vi "LabVIEWRTControlStartupVI.vi"() -> ()   [LabVIEW 2020]
doc: "This example demonstrates a command based communication architecture using TCP. It shows a protocol for packaging and parsing data while minimizing network traffic. Refer to the National Instruments Web site at ni.com/info and enter the info code \"commtcp\" for more information about this command based communication architecture."
uses:
  Control 2.ctl
  ChannelCommand.ctl
  Control 1.ctl
  WaveType.ctl
  MoterEnable.ctl
  <instrlib>/vmic5565/labview-user.lib/VMIC/VMIC 5565 Reflective Memory.llb/VMIC Reference.ctl
  <vilib>/Platform/TimedLoop/XDataNode/timing_clust.ctl
  <vilib>/Platform/TimedLoop/XDataNode/nitl_modes.ctl
  <vilib>/Platform/TimedLoop/XDataNode/wakeup.ctl
  <vilib>/DAQmx/write.llb/DAQmx Write (Analog 1D DBL NChan 1Samp).vi
  <vilib>/DAQmx/write.llb/DAQmx Write (Digital 1D Bool NChan 1Samp 1Line).vi
  <instrlib>/vmic5565/labview-user.lib/VMIC/VMIC 5565 Reflective Memory.llb/VMIC Write (U32).vi
  <vilib>/DAQmx/miscellaneous.llb/DAQmx Fill In Error Info.vi
  <instrlib>/vmic5565/labview-user.lib/VMIC/VMIC 5565 Reflective Memory.llb/VMIC Read (U8).vi
  <vilib>/Platform/TimedLoop/XDataNode/XDataNode.xnode
  <vilib>/Platform/TimedLoop/XDataNode/XDNodeRunTimeDep.lvlib
  <vilib>/real-time/NI_Real-Time Libraries.lvlib
  <vilib>/NI_Real-Time Target Support.lvlib
  <vilib>/real-time/rtutility.llb/RT Restart Target (Self).vi
panel:
  out "输出数组":dbl[](array[numeric])
  out "AngleSample":dbl[](array[numeric])
  out "周期":i64
  out "error out 19":errorcluster caption="错误输出"
  out "error out 18":errorcluster caption="错误输出"
  out "error out 17":errorcluster caption="错误输出"
  out "延迟完成？[i-1]":bool
  out "超时":i32
  out "error out 16":errorcluster caption="错误输出"
  out "error out 15":errorcluster caption="错误输出"
  out "error out 14":errorcluster caption="错误输出"
  out "error out 13":errorcluster caption="错误输出"
  out "error out 3":errorcluster caption="错误输出"
  out "dt":dbl
  out "ResetPosition":dbl[](array[numeric])
  out "Protect":bool
  out "error out 12":errorcluster caption="错误输出"
  out "error out 11":errorcluster caption="error out"
  out "error out 10":errorcluster caption="error out"
  out "error out 9":errorcluster caption="error out"
  out "上传数组":dbl[](array[numeric])
  out "VMIC write":sgl[](array[numeric])
  out "6612counterTask 5":refnum<k21>
  out "ResetAforce":dbl[](array[numeric])
  out "6612counterTask 4":refnum<k21>
  out "6612counterTask 3":refnum<k21>
  out "6612counterTask 2":refnum<k21> caption="任务输出"
  out "6612counterTask":refnum<k21>
  out "x与y? 4":bool[](array[boolean])
  out "VMIC reference":T1
  out "PXI6363IO":refnum<k21>
  out "error out 6":errorcluster caption="error out"
  out "error out 4":errorcluster
  out "Command Type":i32
  out "Msg Head":string
  out "error out":errorcluster caption="错误输出"
  out "长度 3":i32
  out "长度 2":i32
  out "长度":i32
  out "connection ID":refnum<k5> caption="连接ID"
  out "6363Task":refnum<k21> caption="任务输出"
  out "加速度信号":dbl[](array[numeric])
  out "轴向力":dbl[](array[numeric])
  out "T_outrange":bool[](array[boolean])
  out "error out 8":errorcluster caption="error out"
  out "error out 7":errorcluster caption="error out"
  out "error out 5":errorcluster caption="错误输出"
  out "TorqueSampledata 2":dbl[](array[numeric])
  out "command out 2":dbl[](array[numeric])
  out "Wave out 2":dbl[](array[numeric])
  out "type out":dbl[](array[numeric])
  out "Enable":bool[](array[boolean])
  out "StartChannelReset":bool[](array[boolean])
  out "retorquedata2":dbl[](array[numeric])
  out "output 4":dbl[](array[numeric])
  out "TestLoops 2":i32
  out "ResetAngle":dbl[](array[numeric])
  out "ResetTorque":dbl[](array[numeric])
  out "error out 2":errorcluster
  in  "Exit":bool
  out "ControlPara":dbl[][](array[numeric])
  out "ChannelSetArray":T2 {"Enable" items=["不使能", "使能"]; "Wave" items=["0指令", "正弦波", "方波", "三角波", "常值", "波形数据", "白噪声", "正弦扫频", "梯度加载", "VMIC"]; "ChannelType" items=["标准波形跟踪"=1, "扫频测试"=2, "消除多余力"=3, "梯度加载"=4, "载荷谱跟踪"=5, "模拟输入跟踪"=9]; "ChannelStatus" items=["通道关", "位置通道", "加载通道"]}
  out "Stop":bool
  out "iCommand":i32
  out "TestLoops":i32
  out "PXI6738DATask":refnum<k21>
  out "Data array":dbl[][](array[numeric])
  out "error  out":errorcluster
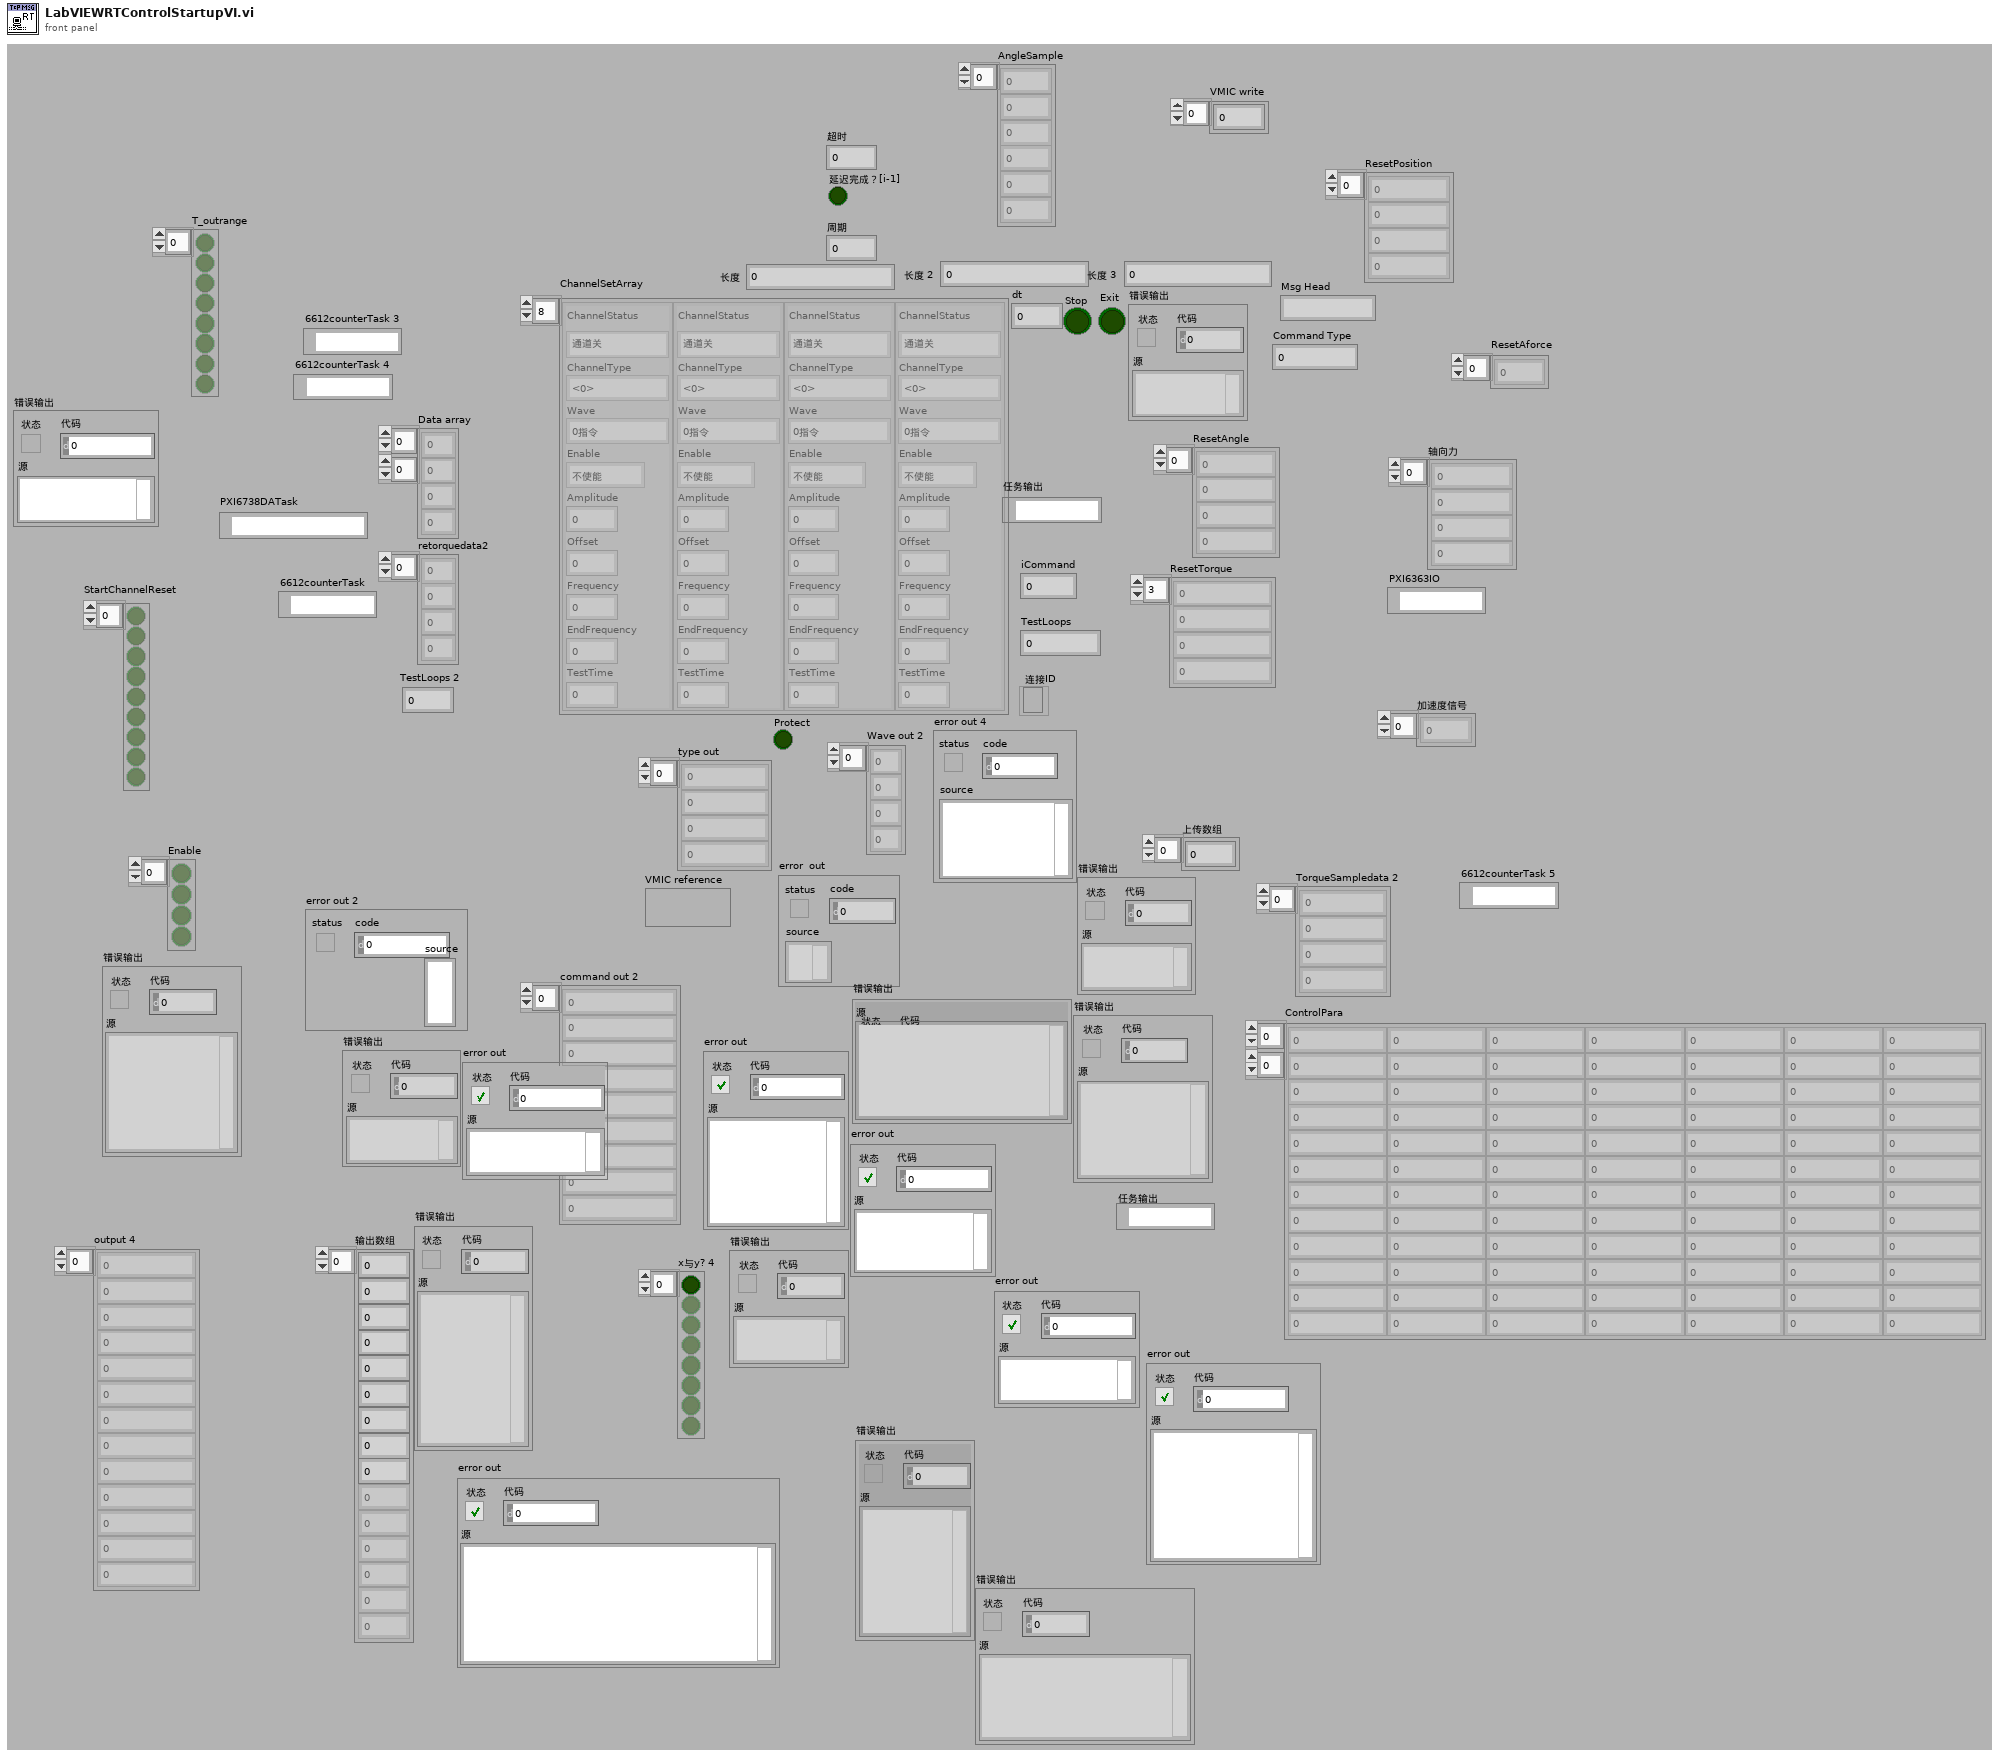
[diagram p1: front panel]
types:
  T1 = typedef "VMIC Reference.ctl" = variant
  T2 = typedef "Control 2.ctl" = T3[]
  T3 = typedef "ChannelCommand.ctl" = cluster{"ChannelStatus":T4, "ChannelType":i32, "Wave":T5, "Enable":T6, "Amplitude":dbl, "Offset":dbl, "Frequency":dbl, "EndFrequency":dbl, "TestTime":dbl}
  T4 = typedef "Control 1.ctl" = i32
  T5 = typedef "WaveType.ctl" = i32
  T6 = typedef "MoterEnable.ctl" = u16
  T7 = typedef "XDNodeRunTimeDep.lvlib/timing_clust.ctl" = cluster{"Expected End [f-1]":u64, "Actual End [f-1]":u64, "Finished Late? [f-1]":bool, "Expected End [i-1]":u64, "Actual End [i-1]":u64, "Finished Late? [i-1]":bool, "Expected Start [i]":u64, "Actual Start [i]":u64, "Expected Start [f]":u64, "Actual Start [f]":u64, "Source Name":string, "Structure Name":string, "Period":i64, "Deadline":i64, "Offset":i64, "Start":i64, "Priority":i32, "Timeout":i32, "Mode":T8, "Wakeup Reason":T9, "Error":errorcluster, "Source Type":string, "Secondary Source Type":string, "Global End Time":u64, "Global Start Time":u64, "Frame Duration":u64, "Iteration Duration":u64, "Assigned CPU":i32, "I/O Scan Engine Mode":u32}
  T8 = typedef "XDNodeRunTimeDep.lvlib/nitl_modes.ctl" = enum32{"No Change", "Process missed periods, maintain original phase", "Discard missed periods, maintain original phase", "Process missed periods, ignore original phase", "Discard missed periods, ignore original phase"}
  T9 = typedef "XDNodeRunTimeDep.lvlib/wakeup.ctl" = enum32{"Normal", "Aborted", "Asynchronous wakeup", "Timing source error", "Timed loop error", "Timeout"}
  T10 = enum16{"big-endian, network order", "native, host order", "little-endian"}
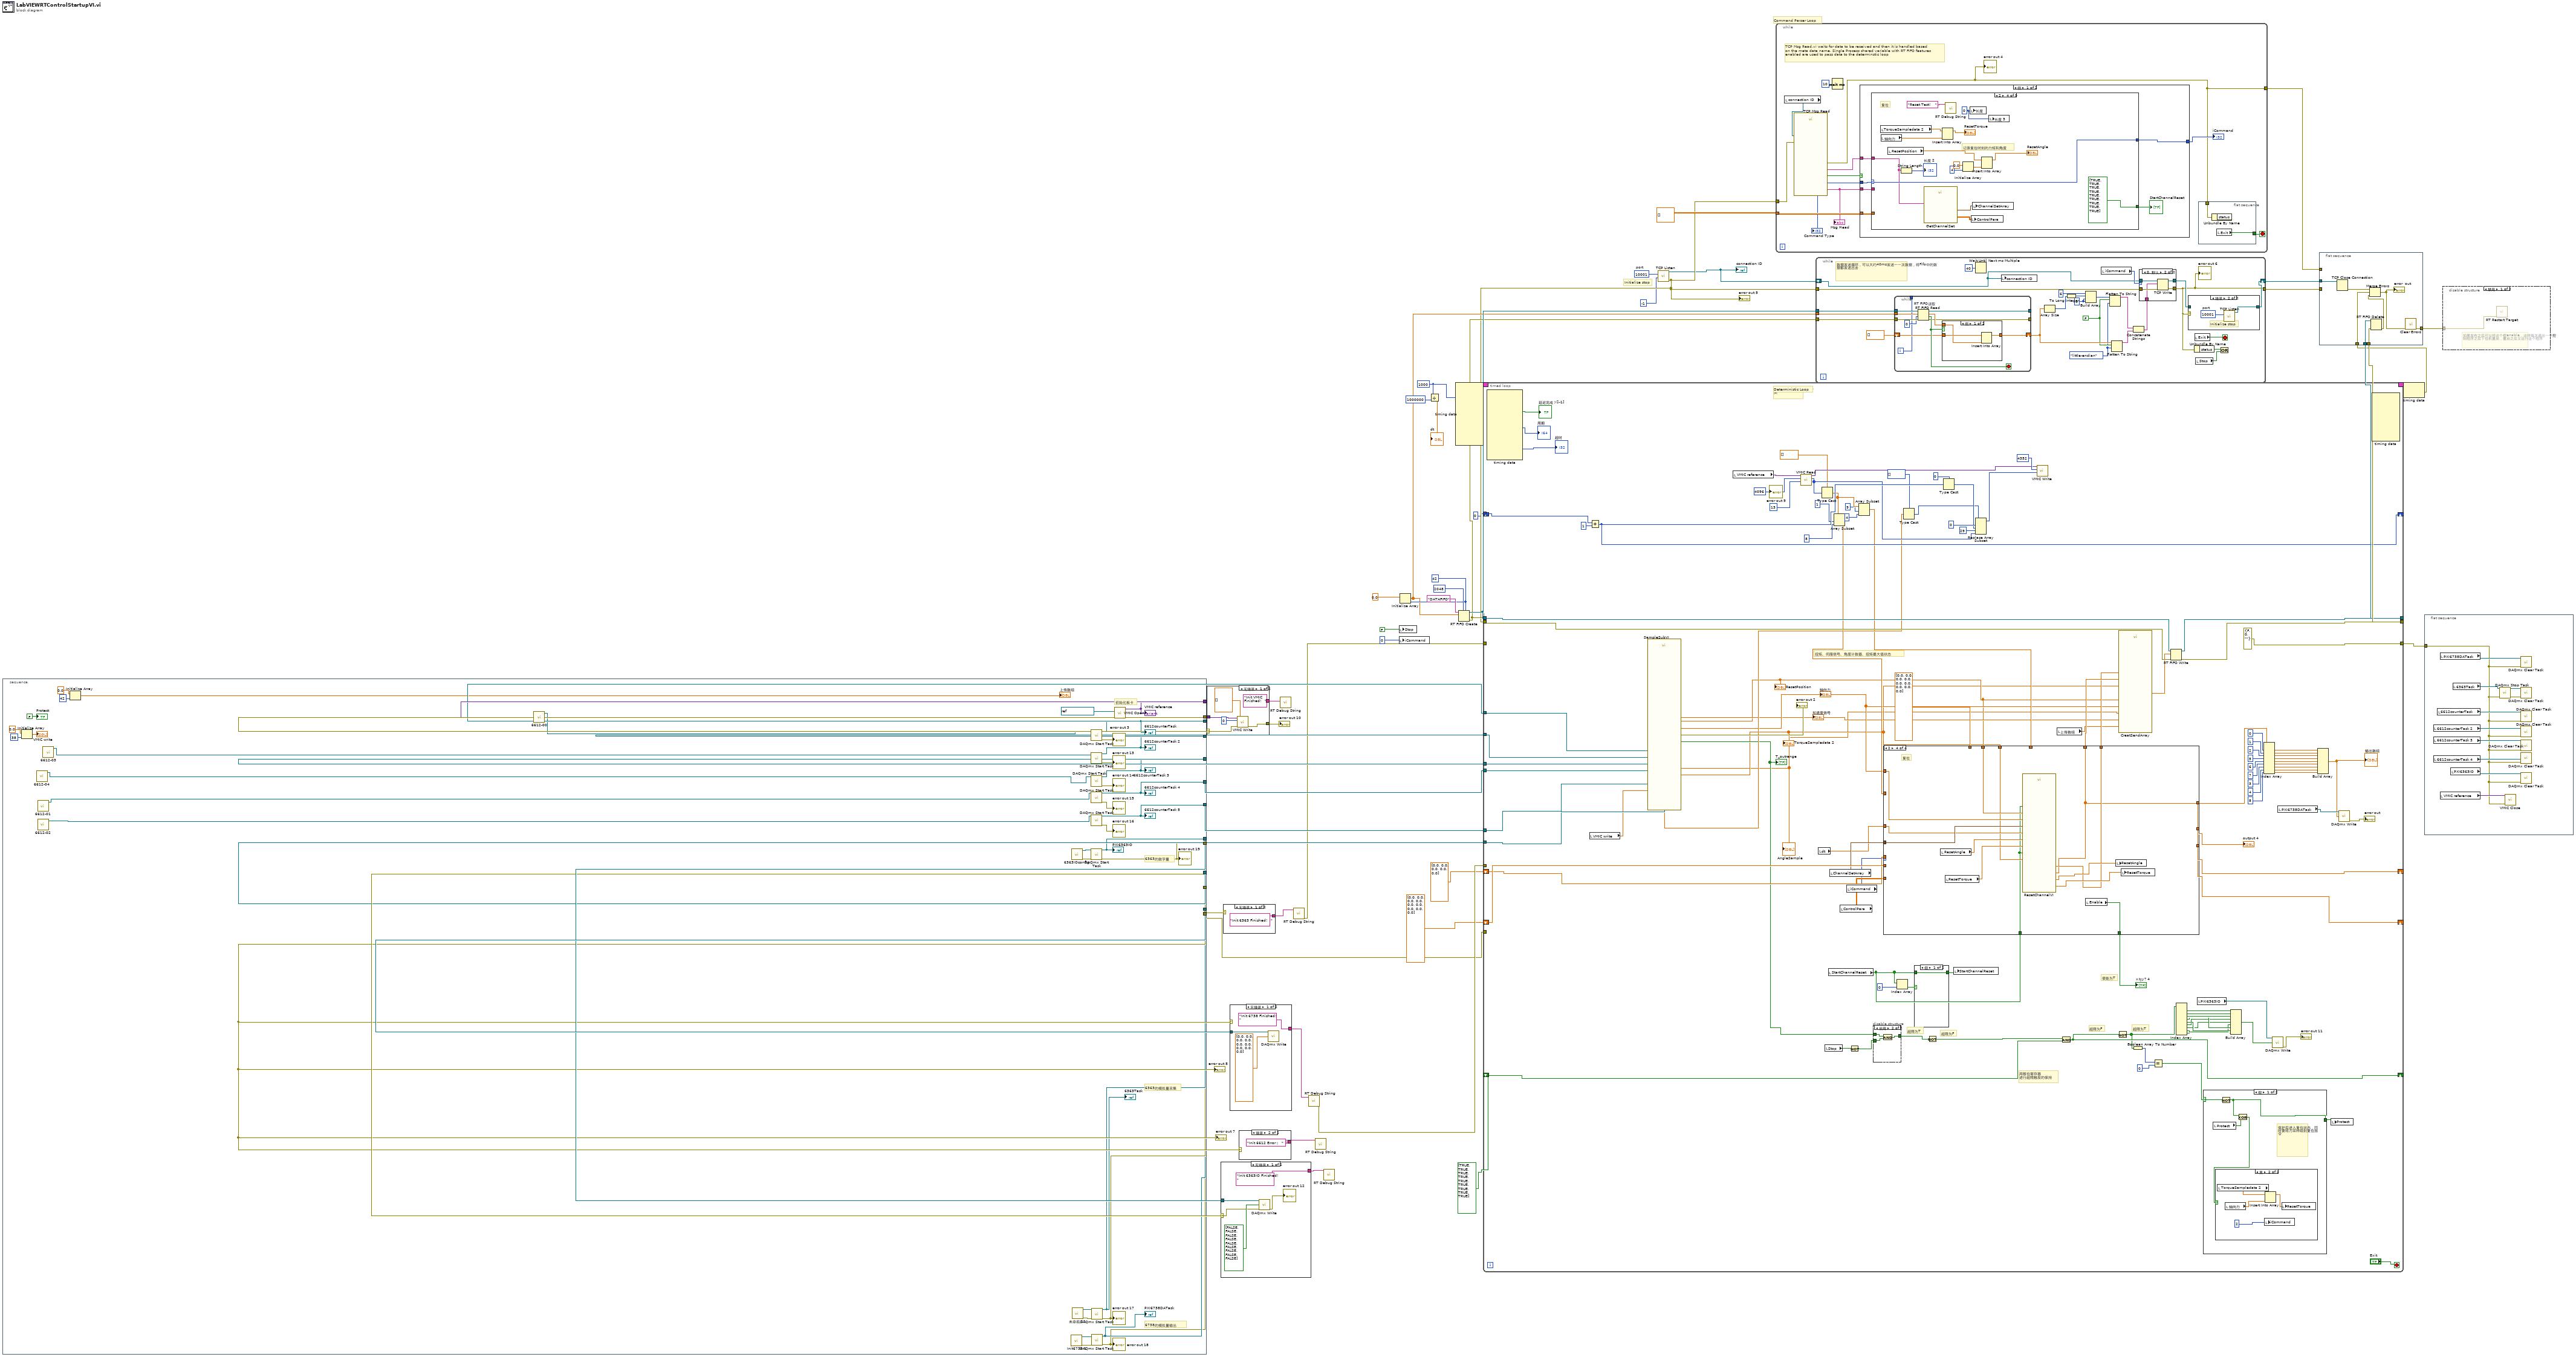
[diagram p0: block diagram]
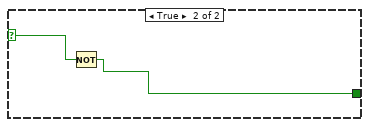
[diagram p3: hidden frame]
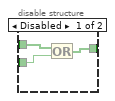
[diagram p4: hidden frame]
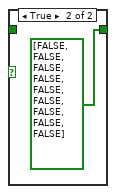
[diagram p5: hidden frame]
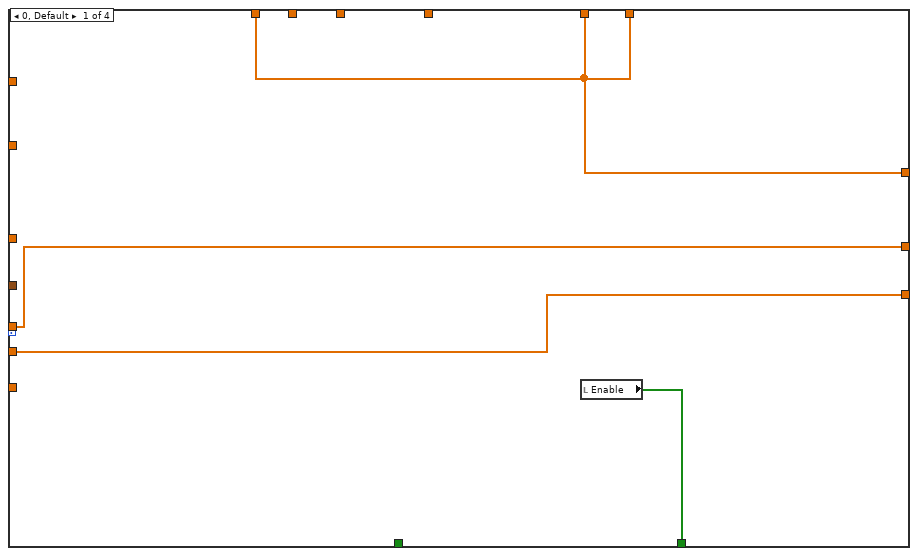
[diagram p6: hidden frame]
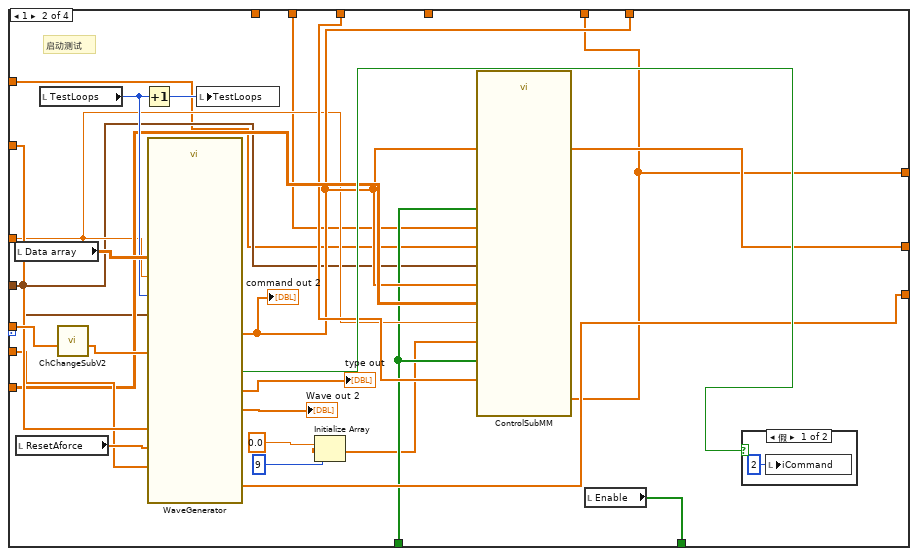
[diagram p7: hidden frame]
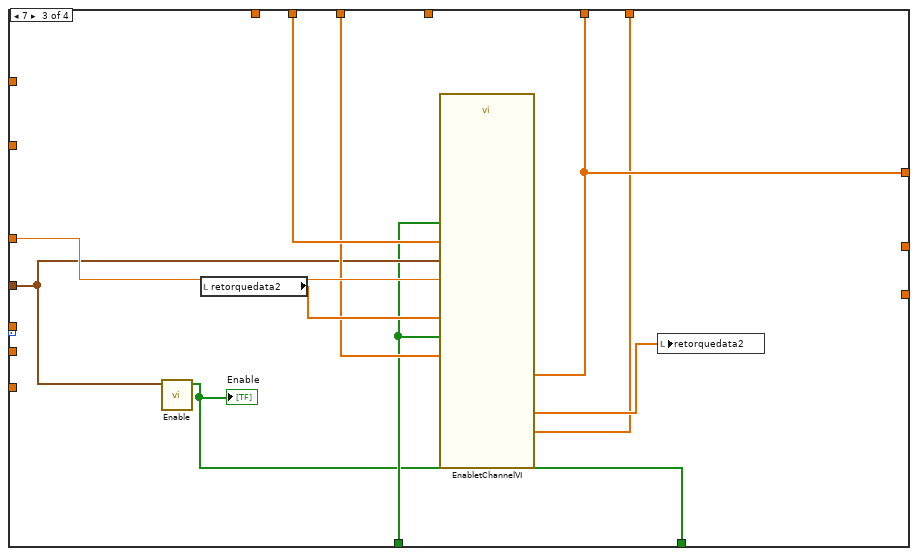
[diagram p9: hidden frame]
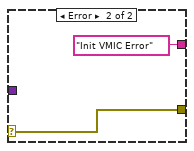
[diagram p10: hidden frame]
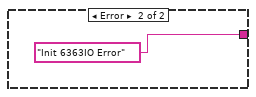
[diagram p11: hidden frame]
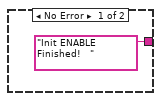
[diagram p12: hidden frame]
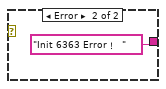
[diagram p13: hidden frame]
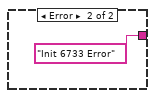
[diagram p15: hidden frame]
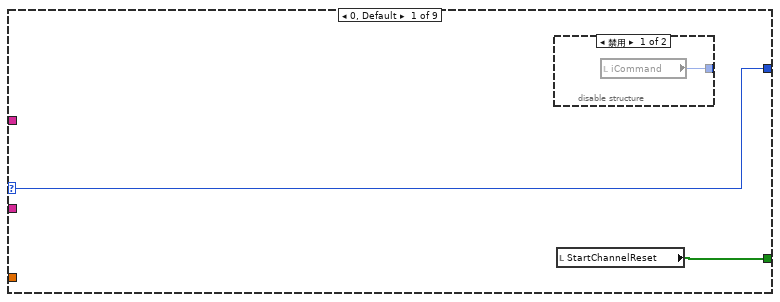
[diagram p16: hidden frame]
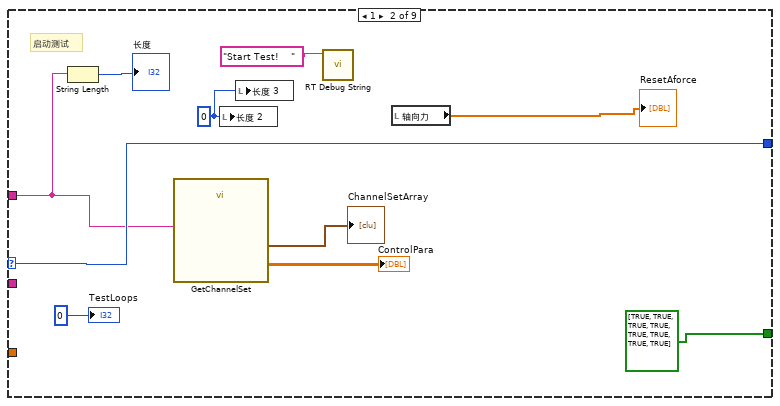
[diagram p18: hidden frame]
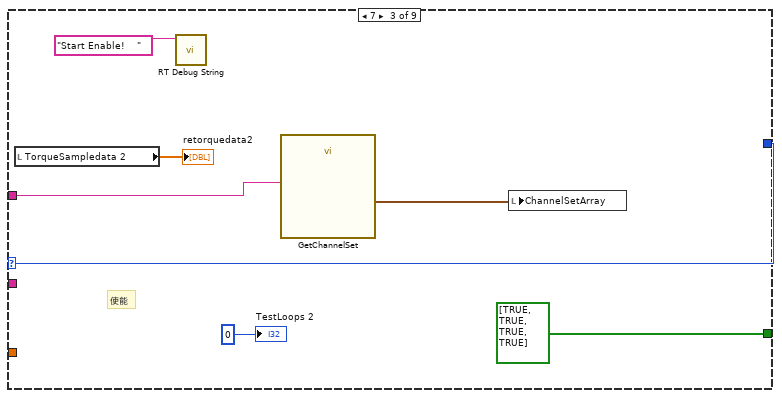
[diagram p19: hidden frame]
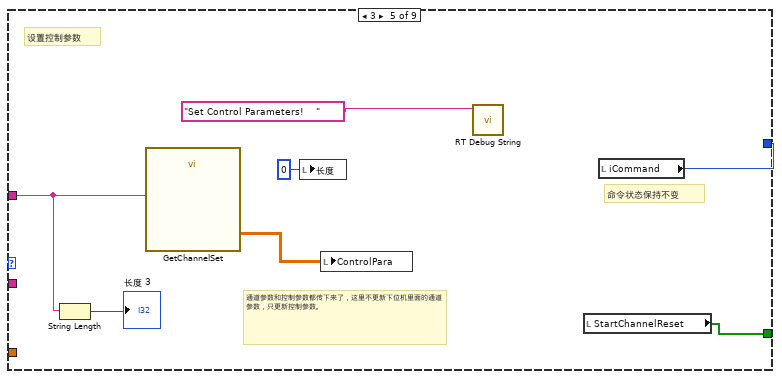
[diagram p20: hidden frame]
diagram:
  w3 = i64 1000 ("周期")
  w46 = u32 42 ("elements in array (1)")
  w52 = u16 10001  # port
  # "Initialize stop"
  # "Command Parser Loop"
  n1 = stacked-sequence {
    tunnel: [w67] -> w9
    tunnel: [w80] -> w28
    tunnel: [w81] -> w10
    tunnel: [w82] -> w11
    tunnel: [w78] -> w24
    tunnel: [w79] -> w26
    tunnel: [w88] -> w23
    tunnel: [w87] -> w22
    tunnel: [w86] -> w20
    tunnel: [w85] -> w19
    tunnel: [w84] -> w18
    tunnel: [w83] -> w17
    tunnel: [w77] -> w16
    frame #0 {
      # "6363的数字量"
      # "6738的模拟量输出"
      # "6363的模拟量采集"
      # "初始化板卡"
      n2 = Initialize Array(sgl 0.0 ("元素"), 38 ("维数大小")) -> (→"VMIC write":sgl[])
      n3 = call "6612-04.vi"() -> ("task out"=w55:refnum<k21>)  [unwired: 10 in, 1 out]
      n4 = call "6612-01.vi"() -> ("task out"=w54:refnum<k21>)  [unwired: 10 in, 1 out]
      n5 = call "6612-02.vi"() -> ("task out"=w53:refnum<k21>)  [unwired: 10 in, 1 out]
      n6 = call "6612-03.vi"() -> ("task out"=w56:refnum<k21>)  [unwired: 10 in, 1 out]
      n7 = Initialize Array(0.0 ("element"), 42 ("dimension size")) -> (→"上传数组":dbl[])
      n8 = call "6612-00.vi"() -> ("task out"=w57:refnum<k21>)  [unwired: 10 in, 1 out]
      n9 = call "Init6738-1.vi"() -> ("error out"=w58:errorcluster, "task out"=w59:refnum<k21>)  [unwired: 10 in]
      n10 = call "6363IOconfig.vi"() -> ("error out"=w60:errorcluster, "task out"=w61:refnum<k21>)  [unwired: 10 in]
      n11 = call "未命名 11.vi"() -> ("error out"=w68:errorcluster, "task out"=w69:refnum<k21>)  [unwired: 10 in]
      n12 = call <vilib>:"DAQmx Start Task.vi"("task/channels in"=w57) -> ("task out"=w86:refnum<k21>, "error out"=→"error out 3":errorcluster)  [unwired: 13 in]
      "6612counterTask" <- w86
      n13 = call <vilib>:"DAQmx Start Task.vi"("task/channels in"=w56) -> ("task out"=w85:refnum<k21>, "error out"=→"error out 13":errorcluster)  [unwired: 13 in]
      "6612counterTask 2" <- w85
      n14 = call <vilib>:"DAQmx Start Task.vi"("task/channels in"=w55) -> ("task out"=w84:refnum<k21>, "error out"=→"error out 14":errorcluster)  [unwired: 13 in]
      "6612counterTask 3" <- w84
      n15 = call <vilib>:"DAQmx Start Task.vi"("task/channels in"=w54) -> ("task out"=w83:refnum<k21>, "error out"=→"error out 15":errorcluster)  [unwired: 13 in]
      "6612counterTask 4" <- w83
      n16 = call <vilib>:"DAQmx Start Task.vi"("task/channels in"=w53) -> ("task out"=w77:refnum<k21>, "error out"=→"error out 16":errorcluster)  [unwired: 13 in]
      "6612counterTask 5" <- w77
      n17 = call <vilib>:"DAQmx Start Task.vi"("task/channels in"=w61, "error in"=w60) -> ("task out"=w79:refnum<k21>, "error out"=w78:errorcluster)  [unwired: 12 in]
      "PXI6363IO" <- w79
      "error out 19" <- w78
      n18 = call <vilib>:"DAQmx Start Task.vi"("task/channels in"=w69, "error in"=w68) -> ("task out"=w82:refnum<k21>, "error out"=w81:errorcluster)  [unwired: 12 in]
      "6363Task" <- w82
      "error out 17" <- w81
      n19 = call <vilib>:"DAQmx Start Task.vi"("task/channels in"=w59, "error in"=w58) -> ("task out"=w80:refnum<k21>, "error out"=w67:errorcluster)  [unwired: 12 in]
      "PXI6738DATask" <- w80
      "error out 18" <- w67
      n20 = call <instrlib>:"VMIC Open.vi"("VISA resource name (empty)"=refnum<visa-resource-name> "PIORC5565") -> ("error out"=w88:errorcluster, "VMIC reference"=w87:T1)  [unwired: 5 in]
      "VMIC reference" <- w87
      "Protect" <- FALSE
    }
  }
  "error out 7" <- w9
  "error out 8" <- w9
  n21 = case shown="无错误" w23 {
    selector: w23 -> [w94 w96]
    tunnel: ["Init VMIC Finished!   " ("String to write") "Init VMIC Error" ("String to write")] -> w21
    tunnel: w22 -> [w91 _]
    tunnel: [w90 w96] -> w13
    frame No Error {
      n22 = call-poly <instrlib>:"VMIC Write.vi"("error in (no error)"=w94, "buffer"=dbl[] [], "offset (0)"=u32 0, "VMIC reference in"=w91) -> ("error out"=w90:errorcluster)  [unwired: 2 in, 1 out]
    }
    frame Error {
    }
  }
  "error out 10" <- w13
  n23 = case shown="无错误" w24 {
    selector: w24 -> [w99 _]
    tunnel: ["Init 6363IO Finished!   " ("String to write") "Init 6363IO Error" ("String to write")] -> w25
    tunnel: w26 -> [w101 _]
    frame No Error {
      n24 = call-poly <vilib>:"DAQmx Write.vi"("task/channels in"=w101, "data"=bool[] [FALSE, FALSE, FALSE, FALSE, FALSE, FALSE, FALSE, FALSE, FALSE], "error in"=w99) -> ("error out"=→"error out 12":errorcluster)  [unwired: 10 in, 2 out]
    }
    frame Error {
    }
  }
  n25 = case shown="无错误" w10 {
    tunnel: ["Init 6363 Finished!   " ("String to write") "Init 6363 Error！  " ("String to write")] -> w38
    frame No Error {
    }
    frame Error {
    }
  }
  n26 = case shown="无错误" w9 {
    tunnel: ["Init 6738 Finished!   " ("String to write") "Init 6733 Error" ("String to write")] -> w36
    tunnel: w28 -> [w106 _]
    frame No Error {
      n27 = call-poly <vilib>:"DAQmx Write.vi"("task/channels in"=w106, "data"=dbl[] [0.0, 0.0, 0.0, 0.0, 0.0, 0.0, 0.0, 0.0, 0.0]) -> ()  [unwired: 11 in, 3 out]
    }
    frame Error {
    }
  }
  n28 = case shown="错误" w9 {
    tunnel: ["Init ENABLE Finished!   " ("String to write") "Init 6612 Error！  " ("String to write")] -> w31
    frame No Error {
    }
    frame Error {
    }
  }
  n29 = call <vilib>:"RT Debug String.vi"("String to write"=w21) -> ()  [unwired: 10 in, 1 out]
  n30 = call <vilib>:"RT Debug String.vi"("String to write"=w38) -> ("error out"=w8:errorcluster)  [unwired: 10 in]
  n31 = call <vilib>:"RT Debug String.vi"("String to write"=w36) -> ("error out"=w37:errorcluster)  [unwired: 10 in]
  n32 = call <vilib>:"RT Debug String.vi"("String to write"=w31) -> ()  [unwired: 10 in, 1 out]
  n33 = call <vilib>:"RT Debug String.vi"("String to write"=w25) -> ()  [unwired: 10 in, 1 out]
  n34 = local write "Stop"(FALSE ("stop")) -> ()
  n35 = local write "iCommand"(0 ("iCommand")) -> ()
  n36 = Initialize Array(0.0, w46) -> (w45:dbl[])
  n37 = Divide(x=w3, y=i64 1000000) -> (x/y=→"dt":dbl)
  n38 = node-c288(w3) -> (w6:T7)  [unwired: 9 in]
  n39 = RT FIFO Create(0:"DATAFIFO" ("name (unnamed)"), 1:w45, 4:u32 2048 ("size (10)"), 6:w46) -> (8:w49:refnum<k33>, 11:w48:errorcluster)  [unwired: 4 in, 1 out]
  n40 = call <vilib>:"TCP Listen.vi"("timeout ms (wait forever: -1)"=-1, "port"=w52) -> ("error out"=w39:errorcluster, "connection ID"=w27:refnum<k5>)  [unwired: 2 in, 6 out]
  "error out 5" <- w39
  "connection ID" <- w27
  n41 = timed-loop {
    tunnel: w48 -> [w221]
    tunnel: w37 -> [_]
    tunnel: w20 -> [w216]
    tunnel: w19 -> [w215]
    tunnel: w18 -> [w214]
    tunnel: w17 -> [w213]
    tunnel: w16 -> [w212]
    tunnel: 0 -> [w210]
    tunnel: w11 -> [w209]
    tunnel: w10 -> [_]
    tunnel: w49 -> [w222]
    tunnel: [w218] -> w32
    tunnel: w39 -> [_]
    tunnel: [w219] -> w33
    tunnel: w8 -> [_]
    tunnel: [errorcluster {"status"=FALSE, "code"=0, "source"=""} ("error in")] -> w40
    shift-right: [w208] -> _
    shift-left: _ -> [_]
    shift-right: [w207] -> _
    shift-left: dbl[] [0.0, 0.0, 0.0, 0.0, 0.0] -> [w211]
    shift-right: [w206] -> _
    shift-left: dbl[] [0.0, 0.0, 0.0, 0.0, 0.0, 0.0, 0.0, 0.0, 0.0] -> [w217]
    shift-right: [w205] -> _
    shift-left: bool[] [TRUE, TRUE, TRUE, TRUE, TRUE, TRUE, TRUE, TRUE, TRUE] -> [w204]
    timing: w6 -> [_]
    timing-out: [_] -> w5
    stop <- "Exit" stop-if-true
    # "用移位寄存器\n进行超限触发的保持"
    # "使能为T"
    # "超限为T"
    # "超限为F"
    # "超限为T"
    # "超限为F"
    # "扭矩、伺服信号、角度计数器、扭矩最大值状态"
    # "将模拟采集通道的数据分类"
    # "Deterministic Loop"
    n42 = node-c288() -> (→"延迟完成？[i-1]":bool, →"周期":i64, →"超时":i32)  [unwired: 1 in, 9 out]
    n43 = local read "VMIC write"() -> (w176:sgl[])
    n44 = Add(x=w210, y=1) -> (x+y=w208:i32)
    n45 = call "SampleSubVI.vi"("task out"=w209, "Courter 1"=w216, "Courter 4"=w213, "Courter 2"=w215, "数组"=w176, "Courter 3"=w214, "Courter 5"=w212) -> ("一级轴向力"=w158:dbl[], "vmic反馈数据"=w177:sgl[], "AngleSample"=w147:dbl[], "加速度信号"=w156:dbl[], "一二级侧向力矩"=w149:dbl[], "F_outrange"=w157:bool[], "error out"=→"error out 2":errorcluster, "一二级侧向位移"=w154:dbl[])  [unwired: 10 in, 3 out]
    "TorqueSampledata 2" <- w149
    "T_outrange" <- w157
    "轴向力" <- w158
    "加速度信号" <- w156
    "ResetPosition" <- w154
    "AngleSample" <- w147
    n46 = local read "VMIC reference"() -> (w170:T1)
    n47 = call-poly <instrlib>:"VMIC Read.vi"("length (0)"=u32 13, "offset (0)"=u32 4096, "VMIC reference in"=w170) -> ("buffer"=w180:u8[], "VMIC reference out"=w174:T1)  [unwired: 2 in, 1 out]
    n48 = local read "dt"() -> (w148:dbl)
    n49 = Type Cast(type=sgl[] [], x=w180) -> (*(type *) &x=w166:sgl[])
    n50 = local read "Stop"() -> (w191:bool)
    n51 = local read "StartChannelReset"() -> (w193:bool[])
    n52 = local read "ChannelSetArray"() -> (w199:T2)
    n53 = Array Subset(array=w166, index=1 ("索引"), length=8 ("长度")) -> (w185:sgl[])
    n54 = local read "ControlPara"() -> (w198:dbl[][])
    n55 = local read "iCommand"() -> (w197:i32)
    n56 = Not(x=w191) -> (.not. x?=w190:bool)
    n57 = Array Subset(array=w166, index=9 ("索引"), length=4 ("长度")) -> (w163:sgl[])
    n58 = disable-structure shown="启用" {
      disable-tunnel: w190 -> [w235 w238]
      disable-tunnel: w157 -> [w234 w237]
      disable-tunnel: [w233 w236] -> w189
      frame Disabled {
        n59 = Or(x=w234, y=w235) -> (x .or. y?=w233:bool[])
      }
      frame Enabled {
        n60 = And(x=w237, y=w238) -> (x .and. y?=w236:bool[])
      }
    }
    n61 = case shown="2" w197 {
      tunnel: [w243 w252 w272 w282] -> w192
      tunnel: [w243 w245 w274 w281] -> w203
      tunnel: dbl[] [0.0, 0.0, 0.0, 0.0, 0.0, 0.0, 0.0, 0.0, 0.0] ("Command") -> [w243 _ _ _]
      tunnel: [w243 w245 w274 w281] -> w131
      tunnel: w154 -> [_ w249 w280 w292]
      tunnel: w149 -> [_ w253 w277 w286]
      tunnel: w199 -> [_ w247 w276 w291]
      tunnel: w148 -> [_ w251 w279 w290]
      tunnel: w198 -> [_ w254 _ _]
      tunnel: w193 -> [_ w250 w273 w285]
      tunnel: [w244 w267 w271 w293] -> w187
      tunnel: w217 -> [w241 w258 _ _]
      tunnel: [w241 w257 _ _] -> w206
      tunnel: [w242 w252 _ _] -> w207
      tunnel: w211 -> [w242 w263 _ _]
      tunnel: w158 -> [_ w246 _ w287]
      tunnel: w185 -> [_ w261 _ _]
      tunnel: w163 -> [_ _ _ _]
      frame 0, Default {
        n62 = local read "Enable"() -> (w244:bool[])
      }
      frame 1 {
        # "启动测试"
        n63 = local read "Data array"() -> (w268:dbl[][])
        n64 = local read "ResetAforce"() -> (w259:dbl[])
        n65 = local read "TestLoops"() -> (w260:i32)
        n66 = call "ChChangeSubV2.vi"("data in"=w263) -> ("data out"=w262:dbl[])  [unwired: 10 in]
        n67 = Increment(x=w260) -> (x+1=w269:i32)
        n68 = call "WaveGenerator.vi"("Data array"=w268, "dt"=w251, "TestLoops"=w260, "VMIC command"=w261, "WaveDefineArray"=w247, "Angle"=w262, "AxisForce"=w259, "LastVMICcommand"=w258) -> ("wave out 2"=→"Wave out 2":dbl[], "Command"=w252:dbl[], "Boolean"=w266:bool, "VMICafterFilter"=w257:dbl[], "type out"=→"type out":dbl[])  [unwired: 3 in]
        "command out 2" <- w252
        n69 = local write "TestLoops"(w269) -> ()
        n70 = Initialize Array(0.0 ("元素"), 9 ("维数大小")) -> (w248:dbl[])
        n71 = call "ControlSubMM.vi"("ControlPara"=w254, "AxisForceSample"=w246, "ChannelSetArray"=w247, "syn-error"=w248, "Angel"=w250, "TorqueSample"=w253, "Command"=w252, "dt"=w251, "Torque"=w250, "AngleSample"=w249) -> ("数组"=w245:dbl[])  [unwired: 5 in]
        n72 = local read "Enable"() -> (w267:bool[])
        n73 = case shown="假" w266 {
          frame False {
            n74 = local write "iCommand"(2 ("iCommand")) -> ()
          }
          frame True {
          }
        }
      }
      frame 7 {
        n75 = call "Enable.vi"("ChannelSetArray2"=w276) -> ("Enable"=w271:bool[])  [unwired: 10 in]
        "Enable" <- w271
        n76 = local read "retorquedata2"() -> (w278:dbl[])
        n77 = call "EnabletChannelVI.vi"("Angelsample"=w280, "Angel"=w273, "dt"=w279, "Torquesample"=w277, "Torque"=w273, "ResetTorqueCommand"=w278, "ChannelSetArray"=w276) -> ("ControlOutput"=w274:dbl[], "ResetTorque 2"=w275:dbl[], "Commandout"=w272:dbl[])  [unwired: 5 in, 1 out]
        n78 = local write "retorquedata2"(w275) -> ()
      }
      frame 2 {
        # "复位"
        n79 = local read "ResetAngle"() -> (w289:dbl[])
        n80 = local read "ResetTorque"() -> (w288:dbl[])
        n81 = call "ResetChannelVI.vi"("Angelsample"=w292, "Angel"=w285, "dt"=w290, "Torquesample"=w286, "Torque"=w285, "ResetAngel"=w289, "ResetTorqueCommand"=w288, "ChannelSetArray"=w291, "AxisForceSample"=w287) -> ("ControlOutput"=w281:dbl[], "resetAngel 2"=w283:dbl[], "ResetTorque 2"=w284:dbl[], "Commandout"=w282:dbl[])  [unwired: 3 in]
        n82 = local read "Enable"() -> (w293:bool[])
        n83 = local write "ResetAngle"(w283) -> ()
        n84 = local write "ResetTorque"(w284) -> ()
      }
    }
    "output 4" <- w131
    "x与y? 4" <- w187
    n85 = Index Array(array=w193, index=0) -> (element=w196:bool)
    n86 = Type Cast(type=u32[] [], x=w177) -> (*(type *) &x=w179:u32[])
    n87 = case shown="假" w196 {
      tunnel: [w239 bool[] [FALSE, FALSE, FALSE, FALSE, FALSE, FALSE, FALSE, FALSE, FALSE]] -> w194
      tunnel: w193 -> [w239 _]
      frame False {
      }
      frame True {
      }
    }
    n88 = Not(x=w189) -> (.not. x?=w188:bool[])
    n89 = Type Cast(type=u32 0, x=w208) -> (*(type *) &x=w182:u32)
    n90 = local write "StartChannelReset"(w194) -> ()
    n91 = Replace Array Subset(array=w179, new element #1=w182, index #1=0 ("索引"), new element #2=w180, index #2=29 ("索引")) -> (w173:u32[])
    n92 = call-poly <instrlib>:"VMIC Write.vi"("buffer"=w173, "offset (0)"=u32 4352, "VMIC reference in"=w174) -> ()  [unwired: 3 in, 2 out]
    n93 = local read "上传数组"() -> (w155:dbl[])
    n94 = And(x=w188, y=w204) -> (x .and. y?=w205:bool[])
    n95 = Not(x=w205) -> (.not. x?=w137:bool[])
    n96 = call "CreatSendArray.vi"("AngleSample"=w147, "AxisForces"=w158, "AccumulateSample"=w156, "数组"=w155, "DisplacementSample"=w154, "ControlOutput"=w203, "TorqueSampledata"=w149, "Command"=w192) -> ("SendArray"=w202:dbl[])  [unwired: 3 in]
    n97 = Boolean Array To Number(Boolean array=w137) -> (number=w161:u32)
    n98 = Equal?(x=w161, y=u32 0) -> (x = y?=w159:bool)
    n99 = RT FIFO Write(0:w222, 1:w202, 3:w221) -> (8:w218:refnum<k33>, 11:w219:errorcluster)  [unwired: 2 in, 2 out]
    n100 = Index Array(array=w137) -> (element #1=w146:bool, element #2=w145:bool, element #3=w144:bool, element #4=w143:bool, element #5=w142:bool, element #6=w141:bool, element #7=w140:bool, element #8=w139:bool, element #9=w138:bool)  [unwired: 9 in]
    n101 = local read "PXI6363IO"() -> (w151:refnum<k21>)
    n102 = case shown="假" w159 {
      selector: w159 -> [w225 w232]
      tunnel: [w223 w231] -> w153
      frame False {
        # "保护后进入复位状态，同时要将力采样给到复位指令"
        n103 = local read "Protect"() -> (w226:bool)
        n104 = Not(x=w225) -> (.not. x?=w223:bool)
        n105 = Exclusive Or(1:w226, 2:w223) -> (0:w224:bool)
        n106 = case shown="真" w224 {
          frame False {
          }
          frame True {
            n107 = local read "TorqueSampledata 2"() -> (w229:dbl[])
            n108 = local read "轴向力"() -> (w230:dbl[])
            n109 = local write "iCommand"(2 ("iCommand")) -> ()
            n110 = Insert Into Array(array=w229, new element=w230) -> (w228:dbl[])  [unwired: 1 in]
            n111 = local write "ResetTorque"(w228) -> ()
          }
        }
      }
      frame True {
        n112 = Not(x=w232) -> (.not. x?=w231:bool)
      }
    }
    n113 = Build Array(w146, w145, w144, w141, w140, w139, w143, w142, w138) -> (w136:bool[])
    n114 = Index Array(array=w131, index #1=0 ("索引"), index #2=1 ("索引"), index #3=2 ("索引"), index #4=5 ("索引"), index #5=6 ("索引"), index #6=7 ("索引"), index #7=3 ("索引"), index #8=4 ("索引"), index #9=8 ("索引")) -> (element #1=w121:dbl, element #2=w120:dbl, element #3=w119:dbl, element #4=w118:dbl, element #5=w117:dbl, element #6=w116:dbl, element #7=w115:dbl, element #8=w114:dbl, element #9=w113:dbl)
    n115 = call-poly <vilib>:"DAQmx Write.vi"("task/channels in"=w151, "data"=w136) -> ("error out"=→"error out 11":errorcluster)  [unwired: 11 in, 2 out]
    n116 = local read "PXI6738DATask"() -> (w132:refnum<k21>)
    n117 = Build Array(w121, w120, w119, w118, w117, w116, w115, w114, w113) -> (w112:dbl[])
    "输出数组" <- w112
    n118 = local write "Protect"(w153) -> ()
    n119 = call-poly <vilib>:"DAQmx Write.vi"("task/channels in"=w132, "data"=w112) -> ("error out"=→"error out":errorcluster)  [unwired: 11 in, 2 out]
    n120 = node-c288() -> ()  [unwired: 8 in, 1 out]
  }
  n121 = while {
    tunnel: w39 -> [w309]
    tunnel: [w302] -> w34
    tunnel: dbl[][] [] -> [w306]
    stop <- w301 stop-if-true
    # "TCP Msg Read.vi waits for data to be received and then it is handled based \non the meta data name. Single Process shared variable with RT FIFO features \nenabled are used to pass data to the determinstic loop"
    n122 = local read "connection ID"() -> (w299:refnum<k5>)
    n123 = call "TCP Msg Read.vi"("connection ID"=w299, "error in"=w309) -> ("Timed Out?"=w308:bool, "Command Type"=w304:i32, "Msg Data"=w307:string, "Msg Head"=w305:string, "error out"=w302:errorcluster)  [unwired: 12 in, 1 out]
    "Msg Head" <- w305
    "Command Type" <- w304
    "error out 4" <- w302
    n124 = Wait (ms)(milliseconds to wait=u32 10 ("等待时间（毫秒）")) -> ()  [unwired: 1 out]
    n125 = case shown="假" w308 {
      tunnel: w307 -> [w317 _]
      tunnel: w304 -> [w316 _]
      tunnel: w306 -> [w315 _]
      tunnel: w305 -> [w314 _]
      tunnel: [w313 w378] -> w303
      frame False {
        n126 = case shown="2" w316 {
          selector: w316 -> [w319 w326 w334 w352 _ w362 w372 w374 _]
          tunnel: w317 -> [_ w324 w337 w346 w355 w369 _ _ _]
          tunnel: w315 -> [_ _ _ _ _ w368 _ _ _]
          tunnel: w314 -> [_ _ _ _ _ w363 _ _ _]
          tunnel: [w319 w326 w334 w352 w358 w362 w372 w374 w377] -> w313
          tunnel: [w318 bool[] [TRUE, TRUE, TRUE, TRUE, TRUE, TRUE, TRUE, TRUE] bool[] [TRUE, TRUE, TRUE, TRUE] bool[] [TRUE, TRUE, TRUE, TRUE, TRUE, TRUE, TRUE, TRUE, TRUE] w357 w361 w371 w373 w376] -> w312
          frame 0, Default {
            n127 = disable-structure shown="禁用" {
              disable-tunnel: [w320 _] -> _
              frame Disabled {
                n128 = local read "iCommand"() -> (w320:i32)
              }
              frame Enabled {
              }
            }
            n129 = local read "StartChannelReset"() -> (w318:bool[])
          }
          frame 1 {
            w322 = 0 ("长度 2")
            # "启动测试"
            n130 = String Length(string=w324) -> (length=→"长度":i32)
            n131 = call "GetChannelSet.vi"("Msg Data"=w324) -> ("ControlPara"=→"ControlPara":dbl[][], "ChannelSetArray"=→"ChannelSetArray":T3[])  [unwired: 9 in]
            n132 = local write "长度 2"(w322) -> ()
            n133 = local write "长度 3"(w322) -> ()
            n134 = call <vilib>:"RT Debug String.vi"("String to write"="Start Test!    ") -> ()  [unwired: 10 in, 1 out]
            n135 = local read "轴向力"() -> (→"ResetAforce":dbl[])
            "TestLoops" <- 0 ("TestLoops")
          }
          frame 7 {
            # "使能"
            n136 = local read "TorqueSampledata 2"() -> (→"retorquedata2":dbl[])
            n137 = call <vilib>:"RT Debug String.vi"("String to write"="Start Enable!    ") -> ()  [unwired: 10 in, 1 out]
            n138 = call "GetChannelSet.vi"("Msg Data"=w337) -> ("ChannelSetArray"=w332:T3[])  [unwired: 9 in, 1 out]
            n139 = local write "ChannelSetArray"(w332) -> ()
            "TestLoops 2" <- 0 ("TestLoops")
          }
          frame 2 {
            w343 = 0 ("长度")
            # "记录复位时刻的力矩和角度"
            # "复位"
            n140 = local read "TorqueSampledata 2"() -> (w349:dbl[])
            n141 = local read "轴向力"() -> (w348:dbl[])
            n142 = local read "ResetPosition"() -> (w339:dbl[])
            n143 = String Length(string=w346) -> (length=→"长度 2":i32)
            n144 = call "GetChannelSet.vi"("Msg Data"=w346) -> ("ControlPara"=w344:dbl[][], "ChannelSetArray"=w345:T3[])  [unwired: 9 in]
            n145 = Insert Into Array(array=w349, new element=w348) -> (→"ResetTorque":dbl[])  [unwired: 1 in]
            n146 = call <vilib>:"RT Debug String.vi"("String to write"="Reset Test!    ") -> ()  [unwired: 10 in, 1 out]
            n147 = Initialize Array(0.0 ("元素"), 4 ("维数大小")) -> (w340:dbl[])
            n148 = local write "长度"(w343) -> ()
            n149 = local write "ControlPara"(w344) -> ()
            n150 = local write "ChannelSetArray"(w345) -> ()
            n151 = Insert Into Array(array=w339, new element=w340) -> (→"ResetAngle":dbl[])  [unwired: 1 in]
            n152 = local write "长度 3"(w343) -> ()
          }
          frame 3 {
            # "命令状态保持不变"
            # "通道参数和控制参数都传下来了，这里不更新下位机里面的通道参数，只更新控制参数。"
            # "设置控制参数"
            n153 = String Length(string=w355) -> (length=→"长度 3":i32)
            n154 = call "GetChannelSet.vi"("Msg Data"=w355) -> ("ControlPara"=w360:dbl[][])  [unwired: 9 in, 1 out]
            n155 = local write "长度"(0 ("长度")) -> ()
            n156 = local write "ControlPara"(w360) -> ()
            n157 = call <vilib>:"RT Debug String.vi"("String to write"="Set Control Parameters!    ") -> ()  [unwired: 10 in, 1 out]
            n158 = local read "StartChannelReset"() -> (w357:bool[])
            n159 = local read "iCommand"() -> (w358:i32)
          }
          frame 6 {
            # "波形数据"
            n160 = call "TCP Data Read.vi"("Data"=w369, "Head"=w363) -> ("Data Channel"=w364:i32, "DataArray"=w367:dbl[])  [unwired: 8 in]
            n161 = Replace Array Subset(array=w368, new element=w367, index (row)=w364) -> (→"Data array":dbl[][])  [unwired: 1 in]
            n162 = local read "StartChannelReset"() -> (w361:bool[])
            n163 = disable-structure shown="Disabled" {
              disable-tunnel: [w370 _] -> _
              frame Disabled {
                n164 = local read "iCommand"() -> (w370:i32)
              }
              frame Enabled {
              }
            }
            n165 = call <vilib>:"RT Debug String.vi"("String to write"="Receive Wave Data\\n") -> ()  [unwired: 10 in, 1 out]
          }
          frame 4 {
            # "停止测试"
            n166 = local read "StartChannelReset"() -> (w371:bool[])
          }
          frame -1 {
            # "退出测试"
            n167 = local read "StartChannelReset"() -> (w373:bool[])
            "Stop" <- TRUE
          }
          frame 88 {
            # "看门狗指令"
            n168 = local read "StartChannelReset"() -> (w376:bool[])
            n169 = local read "iCommand"() -> (w377:i32)
          }
        }
        "StartChannelReset" <- w312
      }
      frame True {
        n170 = local read "iCommand"() -> (w378:i32)
      }
    }
    "iCommand" <- w303
    n171 = flat-sequence {
      tunnel: w302 -> [w311]
      tunnel: [w310] -> w301
      frame #0 {
        n172 = Unbundle By Name(w311) -> ()  [unwired: 1 out]
        n173 = local read "Exit"() -> (w310:bool)
      }
    }
  }
  n174 = while {
    tunnel: w39 -> [w401]
    tunnel: [w379] -> w35
    tunnel: w49 -> [w399]
    tunnel: w48 -> [w400]
    tunnel: w45 -> [w398]
    shift-right: [w381] -> w41
    shift-left: w27 -> [w380]
    stop <- w383 stop-if-true
    w386 = 0 ("element")
    w390 = FALSE ("prepend array or string size? (T)")
    w389 = T10."little-endian" ("byte order (0:big-endian, network order)")
    # "数据发送循环，可以大约40ms发送一一次数据，将Fifo中的数据都发送出去"
    n175 = while {
      tunnel: w399 -> [w424]
      tunnel: w400 -> [w423]
      tunnel: w398 -> [w422]
      shift-right: [w415] -> w394
      shift-left: dbl[] [] -> [w416]
      tunnel: [w420] -> _
      tunnel: [w417] -> _
      tunnel: [w414] -> _
      i -> [w414]
      stop <- w419 stop-if-true
      n176 = RT FIFO Read "RT FIFO读取"(0:w424, 1:w422, 2:0 ("timeout in ms (0)"), 3:w423) -> (8:w420:refnum<k33>, 9:w418:dbl[], 10:w419:bool, 11:w417:errorcluster)  [unwired: 1 out]
      n177 = case shown="假" w419 {
        tunnel: w418 -> [w425 _]
        tunnel: w416 -> [w427 w428]
        tunnel: [w426 w428] -> w415
        frame False {
          n178 = Insert Into Array(array=w427, new element=w425) -> (w426:dbl[])  [unwired: 1 in]
        }
        frame True {
        }
      }
    }
    n179 = Wait Until Next ms Multiple(millisecond multiple=u32 40) -> ()  [unwired: 1 out]
    n180 = local write "connection ID"(w380) -> ()
    n181 = Array Size(array=w394) -> (size(s)=w385:i32)
    n182 = To Long Integer(number=w385) -> (32bit integer=w387:i32)
    n183 = Build Array(6 ("data"), w387, w386, w386) -> (w391:i32[])
    n184 = local read "iCommand"() -> (w384:i32)
    n185 = Flatten To String(anything=w391, prepend array or string size? (T)=w390, byte order (0:big-endian, network order)=w389) -> (data string=w388:string)  [unwired: 1 in, 2 out]
    n186 = Flatten To String(anything=w394, prepend array or string size? (T)=w390, byte order (0:big-endian, network order)=w389) -> (data string=w393:string)  [unwired: 1 in, 2 out]
    n187 = Concatenate Strings(w388, w393) -> (w395:string)
    n188 = case shown="0, 默认" w384 {
      tunnel: w380 -> [w408 w413]
      tunnel: [w408 w412] -> w382
      tunnel: [w407 w411] -> w379
      tunnel: w401 -> [w407 w410]
      tunnel: w395 -> [_ w409]
      frame -1 {
      }
      frame 0, Default {
        n189 = TCP Write(connection ID=w413, data in=w409, error in (no error)=w410) -> (connection ID out=w412:refnum<k5>, error out=w411:errorcluster)  [unwired: 1 in, 1 out]
      }
    }
    "error out 6" <- w379
    n190 = case shown="错误" w379 {
      tunnel: w382 -> [w404 _]
      tunnel: [w404 w405] -> w381
      frame No Error {
      }
      frame Error {
        w406 = u16 10001  # port
        # "Initialize stop"
        n191 = call <vilib>:"TCP Listen.vi"("port"=w406) -> ("connection ID"=w405:refnum<k5>)  [unwired: 3 in, 7 out]
      }
    }
    n192 = Unbundle By Name(w379) -> ("status"=w402:bool)
    n193 = local read "Exit"() -> (w383:bool)
    n194 = local read "Stop"() -> (w397:bool)
    n195 = Or(x=w402, y=w397) -> ()  [unwired: 1 out]
  }
  n196 = flat-sequence {
    tunnel: w4 -> [w436]
    tunnel: [w435] -> w30
    tunnel: w41 -> [w434]
    tunnel: w35 -> [_]
    tunnel: w34 -> [_]
    tunnel: w33 -> [w431]
    tunnel: w32 -> [w430]
    frame #0 {
      n197 = TCP Close Connection(connection ID=w434) -> (error out=w433:errorcluster)  [unwired: 1 in, 2 out]
      n198 = RT FIFO Delete(0:w430, 3:w431) -> (11:w429:errorcluster)  [unwired: 1 in]
      n199 = Merge Errors(w433, w436, w429) -> (w432:errorcluster)
      "error  out" <- w432
      n200 = call <vilib>:"Clear Errors.vi"("error in (no error)"=w432) -> ("error out"=w435:errorcluster)  [unwired: 5 in, 1 out]
    }
  }
  n201 = node-c288(w5) -> (w4:errorcluster)
  n202 = flat-sequence {
    tunnel: w40 -> [w437]
    frame #0 {
      n203 = local read "6612counterTask 2"() -> (w442:refnum<k21>)
      n204 = local read "6612counterTask 3"() -> (w441:refnum<k21>)
      n205 = local read "6612counterTask 4"() -> (w440:refnum<k21>)
      n206 = local read "6612counterTask"() -> (w443:refnum<k21>)
      n207 = local read "PXI6738DATask"() -> (w444:refnum<k21>)
      n208 = local read "VMIC reference"() -> (w438:T1)
      n209 = local read "PXI6363IO"() -> (w439:refnum<k21>)
      n210 = local read "6363Task"() -> (w445:refnum<k21>)
      n211 = call <vilib>:"DAQmx Stop Task.vi"("task/channels in"=w445, "error in"=w437) -> ("task out"=w447:refnum<k21>, "error out"=w446:errorcluster)  [unwired: 12 in]
      n212 = call <instrlib>:"VMIC Close.vi"("error in (no error)"=w437, "VMIC reference in"=w438) -> ()  [unwired: 5 in, 1 out]
      n213 = call <vilib>:"DAQmx Clear Task.vi"("task in"=w444, "error in"=w437) -> ()  [unwired: 13 in, 1 out]
      n214 = call <vilib>:"DAQmx Clear Task.vi"("task in"=w447, "error in"=w446) -> ()  [unwired: 13 in, 1 out]
      n215 = call <vilib>:"DAQmx Clear Task.vi"("task in"=w443, "error in"=w437) -> ()  [unwired: 13 in, 1 out]
      n216 = call <vilib>:"DAQmx Clear Task.vi"("task in"=w442, "error in"=w437) -> ()  [unwired: 13 in, 1 out]
      n217 = call <vilib>:"DAQmx Clear Task.vi"("task in"=w441, "error in"=w437) -> ()  [unwired: 13 in, 1 out]
      n218 = call <vilib>:"DAQmx Clear Task.vi"("task in"=w440, "error in"=w437) -> ()  [unwired: 13 in, 1 out]
      n219 = call <vilib>:"DAQmx Clear Task.vi"("task in"=w439, "error in"=w437) -> ()  [unwired: 13 in, 1 out]
    }
  }
  n220 = disable-structure shown="禁用" {
    disable-tunnel: w30 -> [w448 _]
    frame Disabled {
      # "如果发布之后可以将这个框enable，这样每次退出一个控制程序之后下位机重启，重启之后又运行这个程序"
      n221 = call-poly <vilib>:"RT Restart Target.vi"("error in (no error)"=w448) -> ()  [unwired: 10 in, 1 out]
    }
    frame Enabled {
    }
  }
